vi "S2DS_MyErrorHandler.vi"(8 "error in (no error)":errorcluster, 10 "Auto clear?":bool, 11 "Instrument name":string) -> (0 "error out":errorcluster)   [LabVIEW 2025]
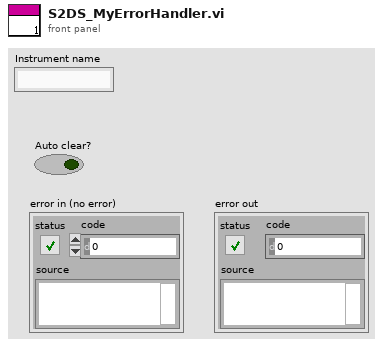
[diagram p1: front panel]
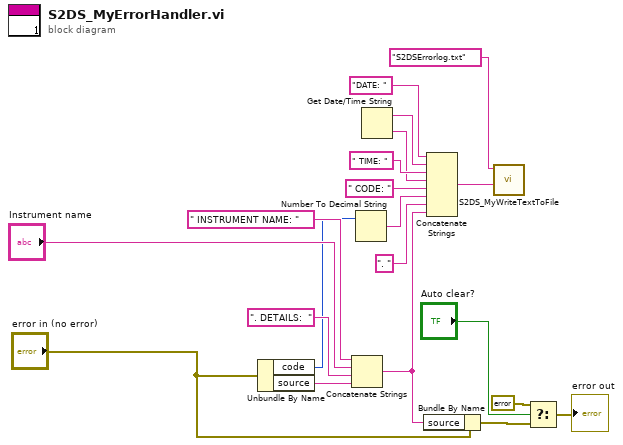
[diagram p0: block diagram]
diagram:
  n1 = Unbundle By Name("error in (no error)") -> ("code"=w10:i32, "source"=w15:string)
  n2 = Concatenate Strings(" INSTRUMENT NAME: " ("string"), "Instrument name", ". DETAILS:  " ("string"), w15) -> (w6:string)
  n3 = Number To Decimal String(number=w10) -> (decimal integer string=w8:string)  [unwired: 1 in]
  n4 = Get Date/Time String() -> (date string=w3:string, time string=w1:string)  [unwired: 3 in]
  n5 = Bundle By Name(cluster="error in (no error)", "source"=w6) -> (w18:errorcluster)
  n6 = Concatenate Strings("DATE: " ("string"), w3, " TIME: " ("string"), w1, " CODE: " ("string"), w8, ". " ("string"), w6) -> (w5:string)
  n7 = call "S2DS_MyWriteTextToFile.vi"("String to write (without line feed)"=w5, "File name"="S2DSErrorlog.txt" ("name or relative path")) -> ()  [unwired: 9 in, 1 out]
  n8 = Select(t=errorcluster {"status"=FALSE, "code"=0, "source"=""}, s="Auto clear?", f=w18) -> (s? t:f=→"error out":errorcluster)
